vi "6. FGV Cnt check.vi"(8 "error in (no error)":errorcluster, 9 "Command":string, 10 "Command type (0 = Normal, 1= ACK, 2 = NACK)":u32, 11 "VISA resource name":refnum<visa-resource-name>="COM3") -> (0 "error out":errorcluster, 1 "Checksum":u32, 3 "Cnt":u32)   [LabVIEW 2014]
uses:
  control/FGV Serial Tasks.ctl
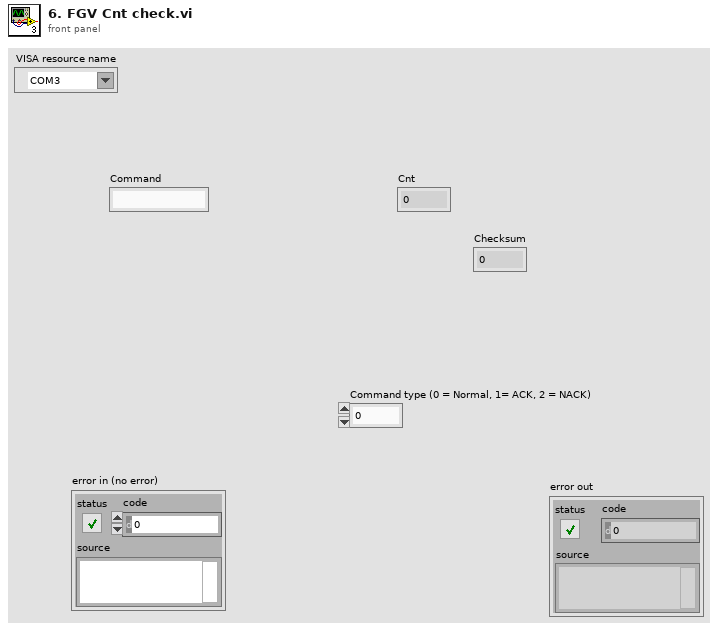
[diagram p1: front panel]
types:
  T1 = typedef "FGV Serial Tasks.ctl" = enum16{"Open", "Read", "Write", "Close", "Flush"}
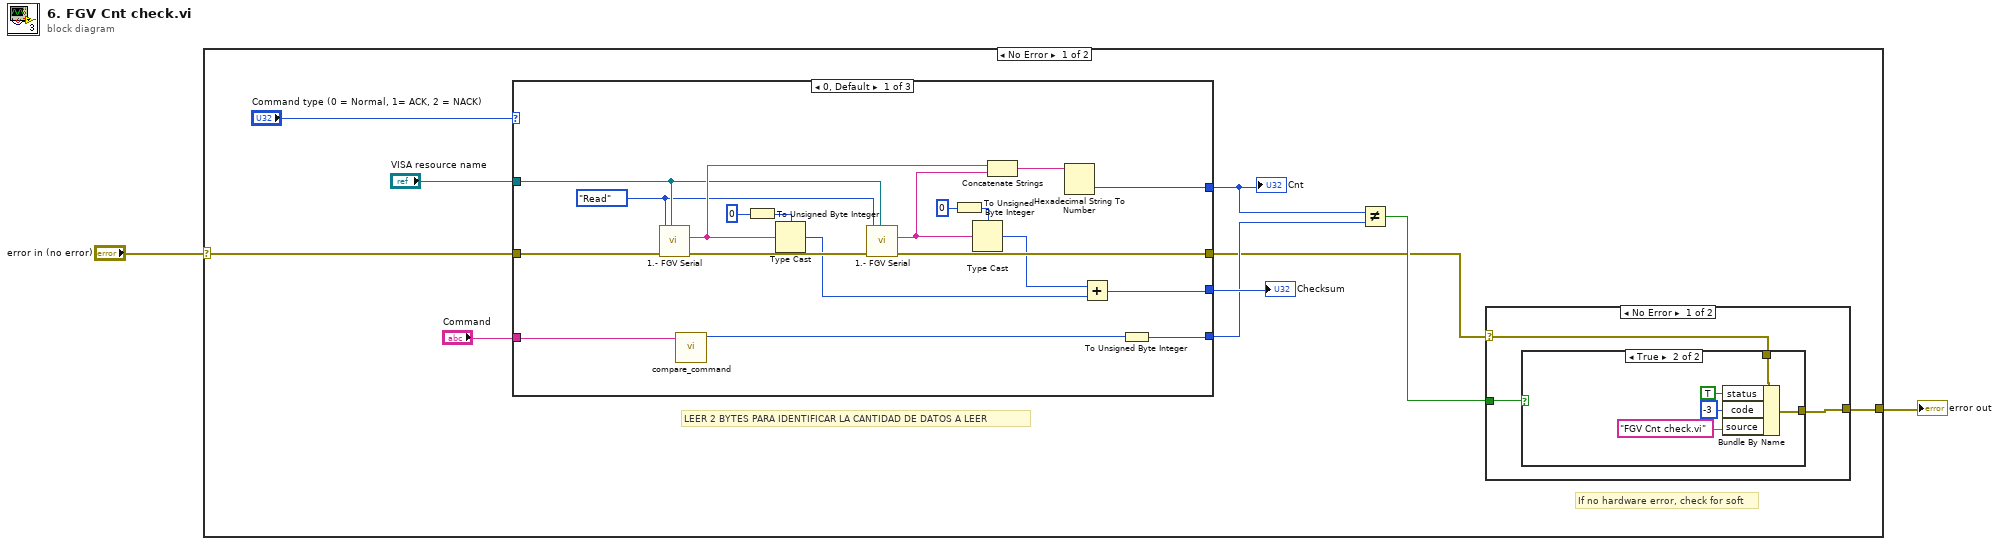
[diagram p0: block diagram]
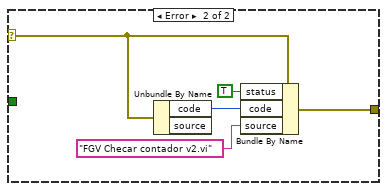
[diagram p3: hidden frame]
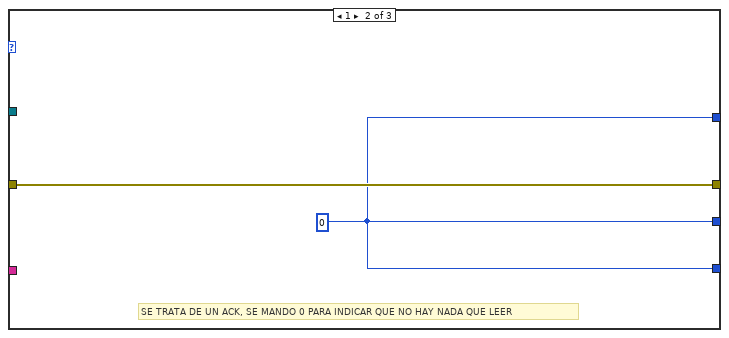
[diagram p4: hidden frame]
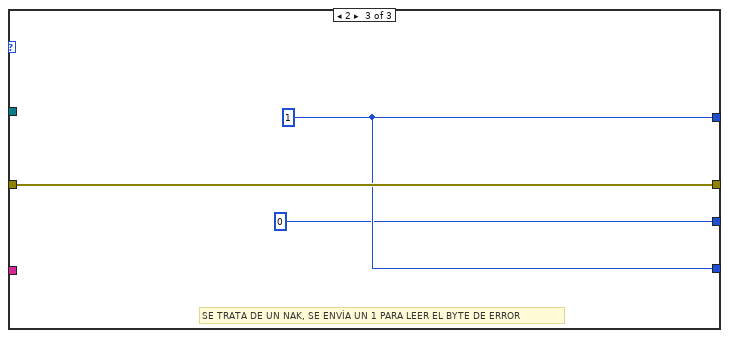
[diagram p5: hidden frame]
diagram:
  n1 = case shown="No Error" "error in (no error)" {
    selector: "error in (no error)" -> [w11 w51]
    tunnel: [w5 w51] -> w1
    frame No Error {
      # "If no hardware error, check for soft"
      # "LEER 2 BYTES PARA IDENTIFICAR LA CANTIDAD DE DATOS A LEER"
      n2 = case shown="0, Default" "Command type (0 = Normal, 1= ACK, 2 = NACK)" {
        tunnel: w11 -> [w45 w47 w50]
        tunnel: [w42 w47 w50] -> w4
        tunnel: [w27 w46 u32 0 ("Checksum")] -> w10
        tunnel: [w40 w46 w49] -> w7
        tunnel: "Command" -> [w39 _ _]
        tunnel: [w37 w46 w49] -> w8
        tunnel: "VISA resource name" -> [w36 _ _]
        frame 0, Default {
          w28 = FGV_Serial_Tasks."Read" ("Task")
          n3 = call "1.- FGV Serial.vi"("VISA resource name"=w36, "error in (no error)"=w45, "Task"=w28) -> ("error out"=w43:errorcluster, "Receive buffer"=w44:string)  [unwired: 6 in, 1 out]
          n4 = call "compare_command.vi"("Command"=w39) -> ("Count"=w38:i32)  [unwired: 9 in, 1 out]
          n5 = To Unsigned Byte Integer(number=u8 0) -> (unsigned 8bit integer=w35:u8)
          n6 = Type Cast(type=w35, x=w44) -> (*(type *) &x=w29:u8)
          n7 = call "1.- FGV Serial.vi"("VISA resource name"=w36, "error in (no error)"=w43, "Task"=w28) -> ("error out"=w42:errorcluster, "Receive buffer"=w31:string)  [unwired: 6 in, 1 out]
          n8 = To Unsigned Byte Integer(number=u8 0) -> (unsigned 8bit integer=w33:u8)
          n9 = Type Cast(type=w33, x=w31) -> (*(type *) &x=w30:u8)
          n10 = Concatenate Strings(w44, w31) -> (w41:string)
          n11 = Hexadecimal String To Number(string=w41) -> (number=w40:u32)  [unwired: 2 in, 1 out]
          n12 = Add(x=w30, y=w29) -> (x+y=w27:u8)
          n13 = To Unsigned Byte Integer(number=w38) -> (unsigned 8bit integer=w37:u8)
        }
        frame 1 {
          w46 = u32 0 ("Checksum")
          # "SE TRATA DE UN ACK, SE MANDO 0 PARA INDICAR QUE NO HAY NADA QUE LEER"
        }
        frame 2 {
          w49 = u32 1 ("Checksum")
          # "SE TRATA DE UN NAK, SE ENVÍA UN 1 PARA LEER EL BYTE DE ERROR"
        }
      }
      "Cnt" <- w7
      "Checksum" <- w10
      n14 = Not Equal?(x=w7, y=w8) -> (x != y?=w6:bool)
      n15 = case shown="No Error" w4 {
        selector: w4 -> [w13 w22]
        tunnel: w6 -> [w15 _]
        tunnel: [w14 w23] -> w5
        frame No Error {
          n16 = case shown="True" w15 {
            tunnel: w13 -> [w16 w21]
            tunnel: [w16 w20] -> w14
            frame False {
            }
            frame True {
              n17 = Bundle By Name(cluster=w21, "status"=TRUE, "code"=-3, "source"="FGV Cnt check.vi") -> (w20:errorcluster)
            }
          }
        }
        frame Error {
          n18 = Unbundle By Name(w22) -> ("code"=w26:i32)  [unwired: 1 out]
          n19 = Bundle By Name(cluster=w22, "status"=TRUE, "code"=w26, "source"="FGV Checar contador v2.vi") -> (w23:errorcluster)
        }
      }
    }
    frame Error {
    }
  }
  "error out" <- w1
